vi "GetAcquisitionDeviceConstants.vi"(11 "key values":T1[](array[typedef])) -> (1 "fpga tach buffer minimum":i32, 2 "fpga tach buffer multiplier":i32, 3 "settling time (seconds)":dbl)   [LabVIEW 2017, in "CmsAcquisition.lvlib"]
uses:
  <vilib>/addons/InsightCM/Devices/Shared/Cms/CmsAcquisition/CmsAcquisition.lvlib
  <vilib>/addons/InsightCM/MessageBus/Base/controls/SectionKeyValues.ctl
  <vilib>/addons/InsightCM/MessageBus/Base/controls/KeyValuePair.ctl
  <vilib>/addons/InsightCM/Utilities/PropertyHelpers/PropertyHelpers.lvlib
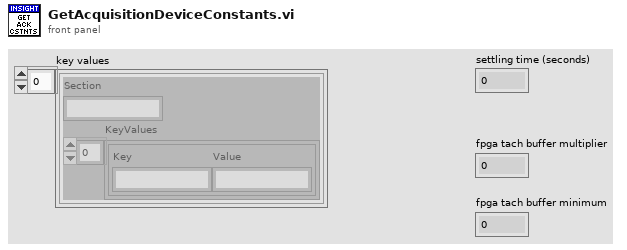
[diagram p1: front panel]
types:
  T1 = typedef "SectionKeyValues.ctl" = cluster{"Section":string, "KeyValues":T2[]}
  T2 = typedef "KeyValuePair.ctl" = cluster{"Key":string, "Value":string}
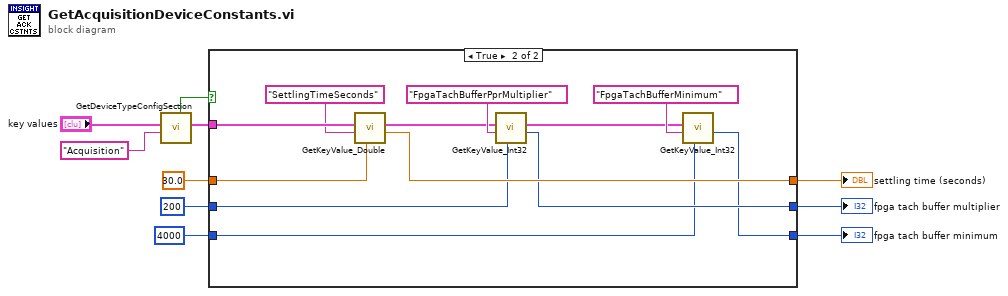
[diagram p0: block diagram]
diagram:
  n1 = call <vilib>:"GetDeviceTypeConfigSection.vi"("key"="Acquisition", "key values"="key values") -> ("key value pairs out"=w7:T2[], "found"=w8:bool)  [unwired: 8 in]
  n2 = case shown="True" w8 {
    tunnel: w7 -> [_ w25]
    tunnel: [w13 w23] -> w6
    tunnel: 30.0 ("value") -> [w13 w22]
    tunnel: 200 ("default") -> [w12 w19]
    tunnel: [w12 w18] -> w3
    tunnel: 4000 ("default") -> [w11 w15]
    tunnel: [w11 w14] -> w1
    frame False {
    }
    frame True {
      n3 = call <vilib>:"GetKeyValue_Double.vi"("default"=w22, "key"="SettlingTimeSeconds" ("Key"), "key value pairs"=w25) -> ("value"=w23:dbl, "key value pairs out"=w20:T2[])  [unwired: 6 in, 1 out]
      n4 = call <vilib>:"GetKeyValue_Int32.vi"("default"=w19, "key"="FpgaTachBufferPprMultiplier" ("Key"), "key value pairs"=w20) -> ("value"=w18:i32, "key value pairs out"=w16:T2[])  [unwired: 6 in, 1 out]
      n5 = call <vilib>:"GetKeyValue_Int32.vi"("default"=w15, "key"="FpgaTachBufferMinimum" ("Key"), "key value pairs"=w16) -> ("value"=w14:i32)  [unwired: 6 in, 2 out]
    }
  }
  "settling time (seconds)" <- w6
  "fpga tach buffer multiplier" <- w3
  "fpga tach buffer minimum" <- w1
